vi "MONTHS.vi"() -> ()   [LabVIEW 2019]
panel:
  in  "MONTH":i32
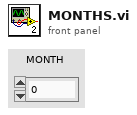
[diagram p1: front panel]
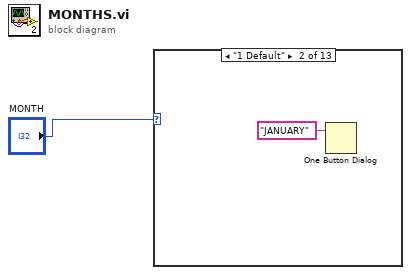
[diagram p0: block diagram]
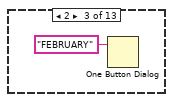
[diagram p3: hidden frame]
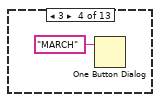
[diagram p4: hidden frame]
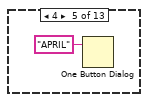
[diagram p5: hidden frame]
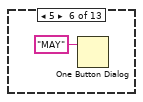
[diagram p6: hidden frame]
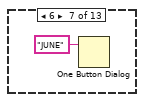
[diagram p7: hidden frame]
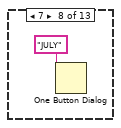
[diagram p8: hidden frame]
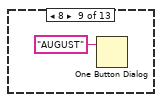
[diagram p9: hidden frame]
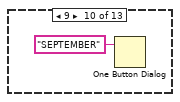
[diagram p10: hidden frame]
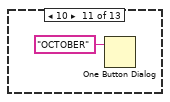
[diagram p11: hidden frame]
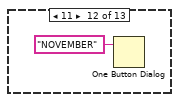
[diagram p12: hidden frame]
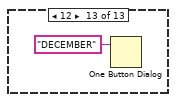
[diagram p13: hidden frame]
diagram:
  n1 = case shown="\"1 Default\"" "MONTH" {
    frame ? {
    }
    frame 0 {
      n2 = One Button Dialog(message="JANUARY") -> ()  [unwired: 1 in, 1 out]
    }
    frame 2 {
      n3 = One Button Dialog(message="FEBRUARY") -> ()  [unwired: 1 in, 1 out]
    }
    frame 3 {
      n4 = One Button Dialog(message="MARCH") -> ()  [unwired: 1 in, 1 out]
    }
    frame 4 {
      n5 = One Button Dialog(message="APRIL") -> ()  [unwired: 1 in, 1 out]
    }
    frame 5 {
      n6 = One Button Dialog(message="MAY") -> ()  [unwired: 1 in, 1 out]
    }
    frame 6 {
      n7 = One Button Dialog(message="JUNE") -> ()  [unwired: 1 in, 1 out]
    }
    frame 7 {
      n8 = One Button Dialog(message="JULY") -> ()  [unwired: 1 in, 1 out]
    }
    frame 8 {
      n9 = One Button Dialog(message="AUGUST") -> ()  [unwired: 1 in, 1 out]
    }
    frame 9 {
      n10 = One Button Dialog(message="SEPTEMBER") -> ()  [unwired: 1 in, 1 out]
    }
    frame 10 {
      n11 = One Button Dialog(message="OCTOBER") -> ()  [unwired: 1 in, 1 out]
    }
    frame 11 {
      n12 = One Button Dialog(message="NOVEMBER") -> ()  [unwired: 1 in, 1 out]
    }
    frame 12 {
      n13 = One Button Dialog(message="DECEMBER") -> ()  [unwired: 1 in, 1 out]
    }
  }
